vi "Send.vi"(8 "error in (no error)":errorcluster, 10 "Message":refnum<class "MSG.lvclass">, 11 "MSR Parent in":refnum<class "MGR.lvclass">) -> (0 "error out":errorcluster, 3 "MSR Parent out":refnum<class "MGR.lvclass">)   [LabVIEW 2011, in "Messenging.lvlib" / "MGR.lvclass"]
uses:
  MGR.lvclass
  Send/Send.lvclass
  SendOnly/Observer.lvclass
  TextVarientMessage/MSG.lvclass
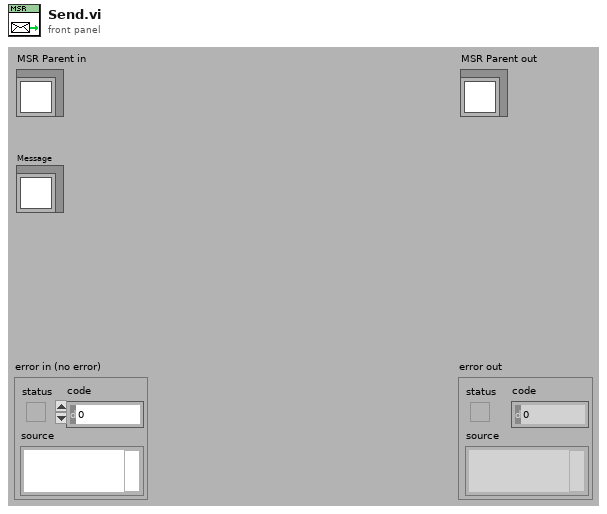
[diagram p1: front panel]
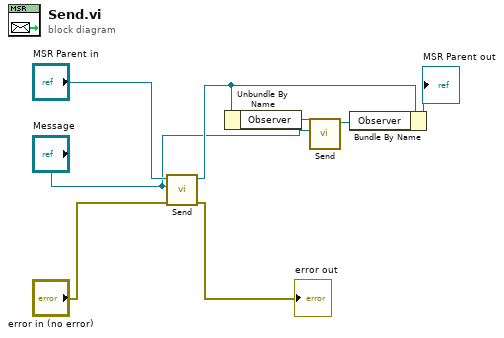
[diagram p0: block diagram]
diagram:
  n1 = call-parent "Send.vi"("error in (no error)"="error in (no error)", "Message"="Message", "MSR Parent in"="MSR Parent in") -> ("error out"=→"error out":errorcluster, "MSR Parent out"=w5:refnum<class "MGR.lvclass">)  [unwired: 7 out]
  n2 = Unbundle By Name(w5) -> ("Observer"=w4:refnum<class "Observer.lvclass">)
  n3 = call-dynamic "Send.vi"("Message"="Message", "MSR Parent in"=w4) -> ("MSR Parent out"=w1:refnum<class "Observer.lvclass">)  [unwired: 1 in, 8 out]
  n4 = Bundle By Name(cluster=w5, "Observer"=w1) -> (→"MSR Parent out":refnum<class "MGR.lvclass">)
